vi "Pkt - Check Packet ID Conflict.vi"(8 "error in (no error)":errorcluster, 10 "New ID":i32, 11 "Packet Ref In":T1=18446744073709551615 format="%.0x") -> (0 "error out":errorcluster, 2 "Conflicting ID?":bool)   [LabVIEW 2016, in "UDP-Custom-Device System Explorer.lvlib"]
uses:
  UDP-Custom-Device System Explorer.lvlib
  <vilib>/NI Veristand/Custom Device API/Custom Device Item Ref.ctl
  <vilib>/NI VeriStand/Custom Device API/Custom Device API.lvlib
  Property Accessors/Shared Packet Accessors.lvlib
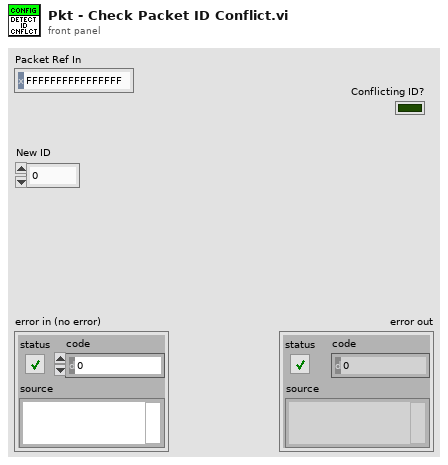
[diagram p1: front panel]
types:
  T1 = typedef "Custom Device API.lvlib/Custom Device Item Ref.ctl" = u64
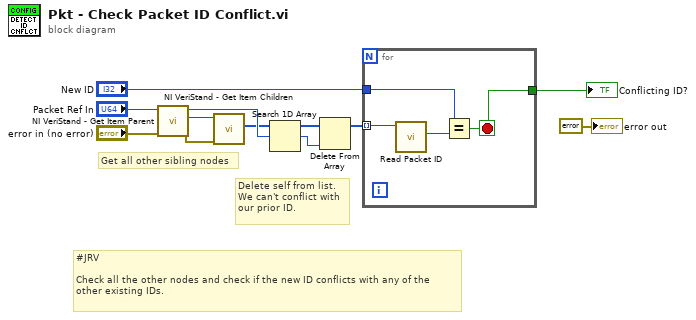
[diagram p0: block diagram]
diagram:
  # "Delete self from list.\nWe can't conflict with\nour prior ID."
  # "Get all other sibling nodes"
  # "#JRV\n\nCheck all the other nodes and check if the new ID conflicts with any of the\nother existing IDs."
  n1 = call <vilib>:"NI VeriStand - Get Item Parent.vi"("error in (no error)"="error in (no error)", "Item Ref in"="Packet Ref In") -> ("error out"=w8:errorcluster, "Parent Ref"=w9:T1, "Item Ref out"=w7:T1)  [unwired: 6 in, 1 out]
  n2 = call <vilib>:"NI VeriStand - Get Item Children.vi"("error in (no error)"=w8, "Item Ref in"=w9) -> ("Child Refs"=w6:T1[])  [unwired: 6 in, 3 out]
  n3 = Search 1D Array(1D array=w6, element=w7) -> (index of element=w5:i32)  [unwired: 1 in]
  n4 = Delete From Array(array=w6, index=w5) -> (array with subset deleted=w4:T1[])  [unwired: 1 in, 1 out]
  n5 = for {
    tunnel: w4 -> [w13] mode=indexing
    tunnel: "New ID" -> [w15]
    tunnel: [w14] -> w2
    stop <- w14 stop-if-true
    n6 = call "Read Packet ID.vi"("Node Ptr"=w13) -> ("Packet ID"=w12:i32)  [unwired: 8 in, 2 out]
    n7 = Equal?(x=w15, y=w12) -> (x = y?=w14:bool)
  }
  "Conflicting ID?" <- w2
  "error out" <- errorcluster {"status"=FALSE, "code"=0, "source"=""} ("error out")
